vi "TagBrowse.vi"(7 "LabVIEW Web Service Request":refnum<class "Web Request.lvclass">) -> ()   [LabVIEW 2013]
uses:
  <vilib>/wsapi/Web Request.lvclass
  <vilib>/NI/Tag Bus Module Framework/channel/TBM channel.lvclass
  <vilib>/NI/TagWebClient/API/String Controls/groupName.ctl
  <vilib>/NI/TagWebClient/API/JSON Formats/TagBrowse Results.ctl
  <vilib>/NI/TagWebClient/API/Logical Groups/Tags in Group.ctl
  <vilib>/NI/TagWebClient/API/String Controls/type.ctl
  <vilib>/NI/TagWebClient/API/Logical Groups/tags.ctl
  <vilib>/NI/TagWebClient/API/String Controls/tagName.ctl
  <vilib>/NI/TagWebClient/API/String Controls/permissions.ctl
  <vilib>/NI/Tag Bus/tag/tag descriptor.lvclass/tag descriptor.ctl
  <vilib>/NI/Tag Bus Module Framework/channel/TBM channel.lvclass/TBM channel.ctl
  <vilib>/NI/Tag Bus/tag/read tag name.vi
  <vilib>/NI/Tag Bus Module Framework/channel/Read channel classification.vi
  <vilib>/NI/Tag Bus/tag/count types.vi
  <vilib>/NI/Tag Bus/tag/index to type.vi
  <vilib>/NI/TagWebClient/API/tagweb client API.lvlib
  <vilib>/NI/Tag Bus/tag/tag descriptor.lvclass
panel:
  # "Use the Web Service Request input terminal to call the VIs on the Web Services palette. Do not remove it from the connector pane unless you don't need access to the palette."
  # "Each additional control wired to the connector pane will be available as an input in the URL. To include an indicator in terminal-mode output (the default setting), it must also be wired to the connector pane."
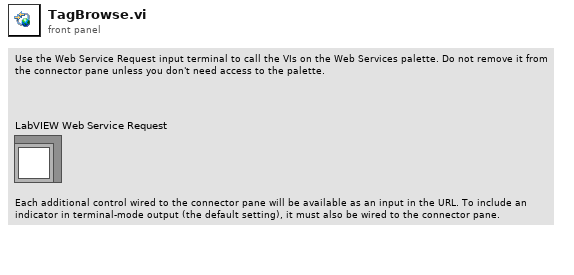
[diagram p1: front panel]
types:
  T1 = typedef "tagweb client API.lvlib/TagBrowse Results.ctl" = cluster{"groupName":T2, "Tags":T3[]}
  T2 = typedef "tagweb client API.lvlib/groupName.ctl" = string
  T3 = typedef "tagweb client API.lvlib/Tags in Group.ctl" = cluster{"type":T4, "tags":T5}
  T4 = typedef "tagweb client API.lvlib/type.ctl" = string
  T5 = typedef "tagweb client API.lvlib/tags.ctl" = cluster{"tagName":T6, "permissions":T7}[]
  T6 = typedef "tagweb client API.lvlib/tagName.ctl" = string
  T7 = typedef "tagweb client API.lvlib/permissions.ctl" = string
  T8 = typedef "tag bus.lvlib/tag descriptor.lvclass/Data Type.ctl" = enum16{"Double", "Single", "I64", "I32", "I16", "I8", "U64", "U32", "U16", "U8", "Boolean", "String", "Array of Double", "Array of Single", "Array of I64", "Array of I32", "Array of I16", "Array of I8", "Array of U64", "Array of U32", "Array of U16", "Array of U8", "Array of Boolean", "Array of String"}
  T9 = typedef "TBM channel.lvclass/channel classification.ctl" = enum16{"input data", "output data", "processing parameter", "processing result"}
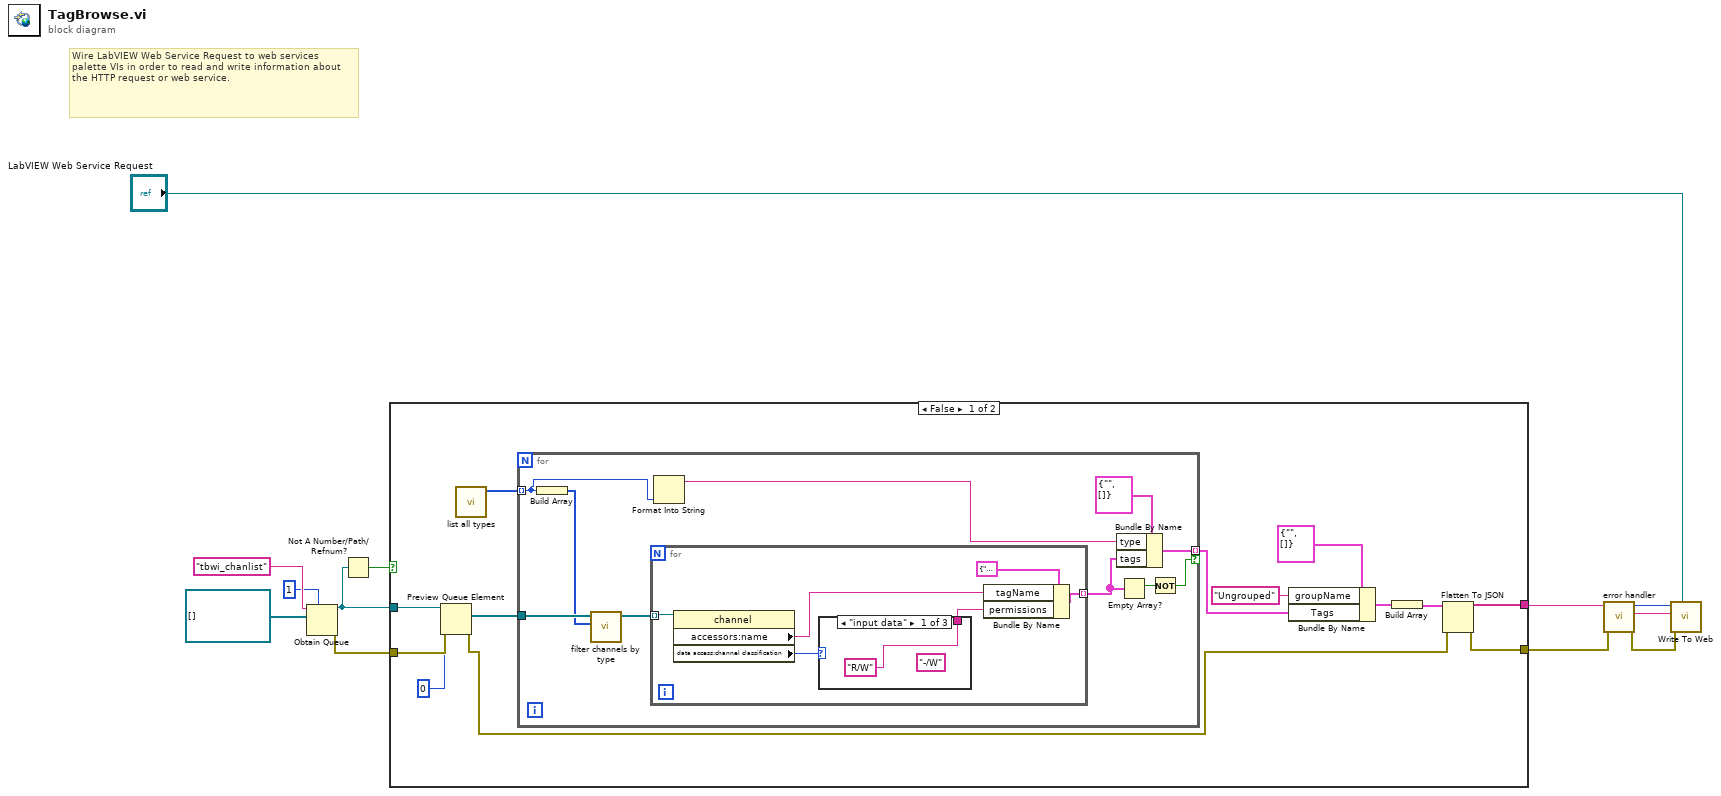
[diagram p0: block diagram]
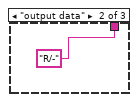
[diagram p2: hidden frame]
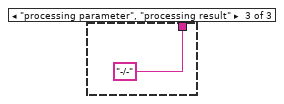
[diagram p3: hidden frame]
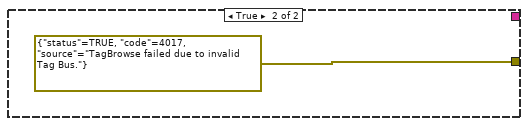
[diagram p4: hidden frame]
diagram:
  # "Wire LabVIEW Web Service Request to web services palette VIs in order to read and write information about the HTTP request or web service."
  n1 = Obtain Queue(max queue size (-1, unlimited)=1, name (unnamed)="tbwi_chanlist", element data type=refnum<class "TBM channel.lvclass">[] [] ("channels in")) -> (queue out=w2:refnum<queue>, error out=w3:errorcluster)  [unwired: 2 in, 1 out]
  n2 = Not A Number/Path/Refnum?(number/path/refnum=w2) -> (NaN/Path/Refnum?=w1:bool)
  n3 = case shown="False" w1 {
    tunnel: w3 -> [w25 _]
    tunnel: w2 -> [w24 _]
    tunnel: [w17 errorcluster {"status"=TRUE, "code"=4017, "source"="TagBrowse failed due to invalid Tag Bus."} ("error out")] -> w12
    tunnel: [w18 _] -> w11
    frame False {
      n4 = Preview Queue Element(queue=w24, timeout in ms (-1)=0, error in (no error)=w25) -> (element=w14:refnum<class "TBM channel.lvclass">[], error out=w16:errorcluster)  [unwired: 2 out]
      n5 = call <vilib>:"list all types.vi"() -> ("all types"=w15:T8[])  [unwired: 11 in]
      n6 = for {
        tunnel: w15 -> [w34] mode=indexing
        tunnel: w14 -> [w31]
        tunnel: [w32] -> w13 mode=indexing if=w26
        n7 = Build Array(w34) -> (w29:T8[])
        n8 = call <vilib>:"filter channels by type.vi"("allowed types"=w29, "channels in"=w31) -> ("channels out"=w30:refnum<class "TBM channel.lvclass">[])  [unwired: 9 in]
        n9 = for {
          tunnel: [w40] -> w28 mode=indexing
          tunnel: w30 -> [w39] mode=indexing
          n10 = property class="channel"(reference=w39) -> ("accessors:name"=w38:string, "data access:channel classification"=w37:T9)  [unwired: 1 in, 2 out]
          n11 = case shown="\"input data\"" w37 {
            tunnel: ["R/W" "R/-" "-/-"] -> w36
            frame "input data" {
              (unwired) "-/W"
            }
            frame "output data" {
            }
            frame "processing parameter", "processing result" {
            }
          }
          n12 = Bundle By Name(cluster=cluster{"tagName":T6, "permissions":T7} {"tagName"="", "permissions"=""} ("Cluster"), "tagName"=w38, "permissions"=w36) -> (w40:cluster{"tagName":T6, "permissions":T7})
        }
        n13 = Format Into String(w34) -> (resulting string=w33:string)  [unwired: 3 in, 1 out]
        n14 = Bundle By Name(cluster=T3 {"type"="", "tags"=[]} ("Cluster"), "type"=w33, "tags"=w28) -> (w32:T3)
        n15 = Empty Array?(array=w28) -> (empty?=w27:bool)
        n16 = Not(x=w27) -> (.not. x?=w26:bool)
      }
      n17 = Bundle By Name(cluster=T1 {"groupName"="", "Tags"=[]} ("Cluster"), "groupName"=T2 "Ungrouped", "Tags"=w13) -> (w21:T1)
      n18 = Build Array(w21) -> (w20:T1[])
      n19 = Flatten To JSON(anything=w20, error in (no error)=w16) -> (JSON string=w18:string, 11:w17:errorcluster)  [unwired: 1 in]
    }
    frame True {
    }
  }
  n20 = call "error handler.vi"("error in (no error)"=w12, "Success Message"=w11) -> ("error out"=w10:errorcluster, "Response String"=w7:string, "Response Code"=w8:i32)  [unwired: 7 in]
  n21 = call <vilib>:"Write To Web.vi"("Web Request in"="LabVIEW Web Service Request", "error in (no error)"=w10, "Response String"=w7, "Response Code"=w8) -> ()  [unwired: 7 in, 1 out]
